vi "priv_Store.UI.Ref.vi"(8 "error in (no error)":errorcluster, 11 "UI_Actor in":refnum<class "UI_Actor.lvclass">) -> (0 "error out":errorcluster, 3 "UI_Actor out":refnum<class "UI_Actor.lvclass">)   [LabVIEW 2020, in "UI_Actor.lvlib" / "UI_Actor.lvclass"]
uses:
  UI_Actor.lvclass
  UI_Actor.lvclass/UI_Actor.ctl
panel:
  # "s'appelle priv mais n'est pas priv car doit etre trig par message,\ndonc peut pas etre priv, mais doit pas etre touché !"
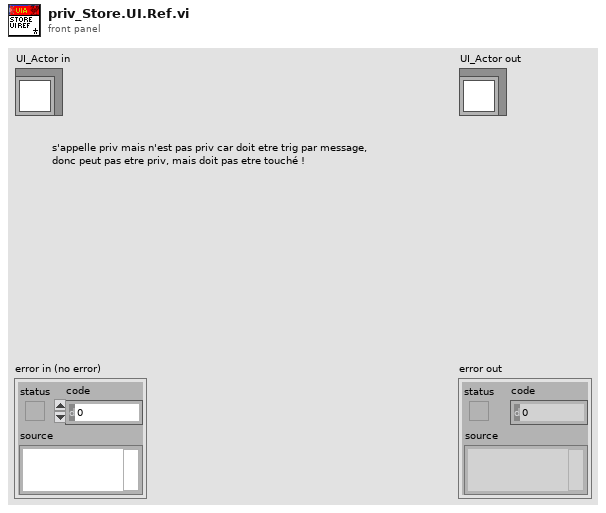
[diagram p1: front panel]
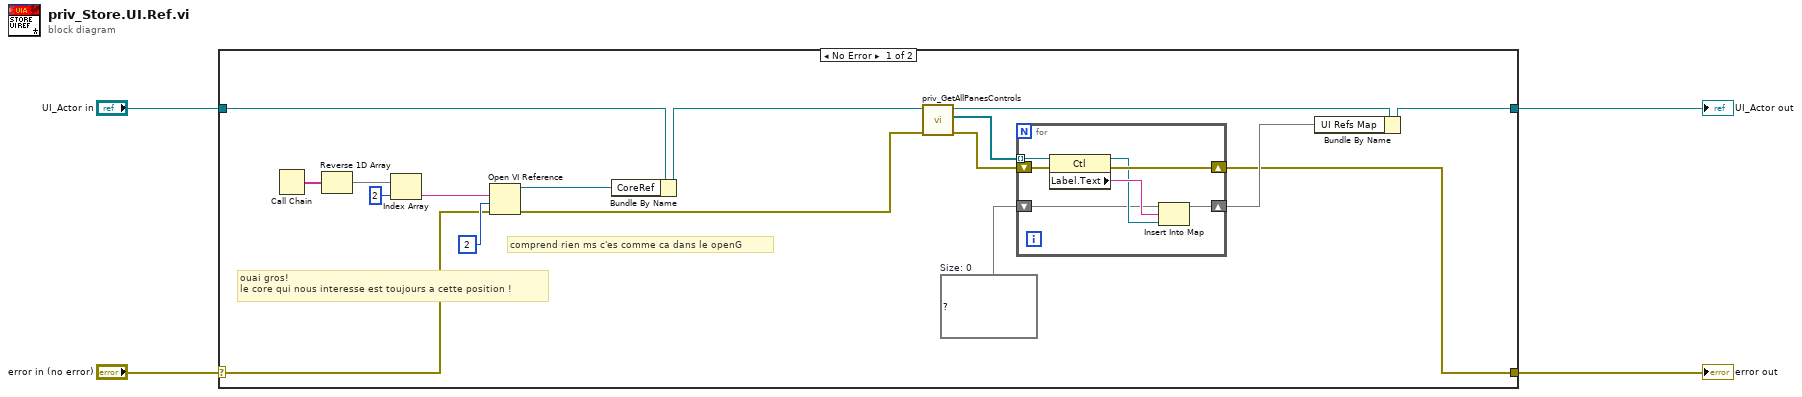
[diagram p0: block diagram]
diagram:
  n1 = case shown="No Error" "error in (no error)" {
    selector: "error in (no error)" -> [w14 w30]
    tunnel: [w5 w30] -> w3
    tunnel: [w10 w29] -> w1
    tunnel: "UI_Actor in" -> [w21 w29]
    frame No Error {
      w11 = map{string, refnum<vi>} {}  # Size: 0
      # "comprend rien ms c'es comme ca dans le openG"
      # "ouai gros!\nle core qui nous interesse est toujours a cette position !"
      n2 = Call Chain() -> (call chain=w20:string[])
      n3 = Reverse 1D Array(array=w20) -> (reversed array=w19:string[])
      n4 = Index Array(array=w19, index=2) -> (element=w16:string)
      n5 = Open VI Reference(vi path=w16, options=2, error in (no error)=w14) -> (vi reference=w15:refnum<vi>, error out=w6:errorcluster)  [unwired: 3 in]
      n6 = Bundle By Name(cluster=w21, "CoreRef"=w15) -> (w8:refnum<class "UI_Actor.lvclass">)
      n7 = call "priv_GetAllPanesControls.vi"("error in (no error)"=w6, "UI_Actor in"=w8) -> ("error out"=w12:errorcluster, "Controls[]"=w13:refnum<vi>[], "UI_Actor out"=w7:refnum<class "UI_Actor.lvclass">)  [unwired: 7 in]
      n8 = for {
        tunnel: w13 -> [w28] mode=indexing
        shift-right: [w26] -> w5
        shift-left: w12 -> [w27]
        shift-right: [w23] -> w9
        shift-left: w11 -> [w22]
        n9 = property class="Ctl"(reference=w28, error in=w27) -> (reference out=w24:refnum<vi>, error out=w26:errorcluster, "Label.Text"=w25:string)
        n10 = Insert Into Map(map in=w22, key=w25, value=w24) -> (map out=w23:map{string, refnum<vi>})  [unwired: 2 out]
      }
      n11 = Bundle By Name(cluster=w7, "UI Refs Map"=w9) -> (w10:refnum<class "UI_Actor.lvclass">)
    }
    frame Error {
    }
  }
  "error out" <- w3
  "UI_Actor out" <- w1
